vi "POST Measurement Details.vi"(0 "GTron in":path, 3 "error in":errorcluster) -> (6 "IsEmpty":bool, 9 "error out":errorcluster)   [LabVIEW 2019, in "DataLogger.lvclass"]
doc: "POST Measurement Details"
uses:
  DataLogger.lvclass
  <vilib>/drjdpowell/SQLite Library/SQL Connection/Execute SQL (Single Integer).vi
  <vilib>/httpClient/LabVIEWHTTPClient.lvlib
  <vilib>/httpClient/POSTBuffer.vi
  <vilib>/drjdpowell/SQLite Library/SQL Connection/Execute SQL (No results).vi
  <vilib>/drjdpowell/SQLite Library/SQL Statement/SQL Statement.lvclass
  <vilib>/drjdpowell/SQLite Library/SQL Connection/Open (path).vi
  <vilib>/drjdpowell/SQLite Library/SQL Connection/Connection.lvclass
panel:
  in  "Server info Cluster for Measurement in":T1={"JSON Buffer"="authtoken=47244d7c61d7e6141acdddeabbf622d1&scope=creatorapi&zc_ownername=zentron3&XMLString=", "Server information start tag"="<ZohoCreator> <applicationlist> <application name='iiot-gtron'><formlist>  <form name='SimulatedMeasurementDetails'>", "Record start/end"="add", "Key name"="field name", "Value name"="value", "Server information end tag"="\"</form></formlist></application></applicationlist></ZohoCreator>"}
  in  "Measurement Keys in":string[](array[string])=["BatchId", "PartName", "MeasurementName", "LSL", "USL", "NominalValue", "LCL", "UCL", "Mean", "StandardDeviation", "Variance", "Cp", "Cpk"]
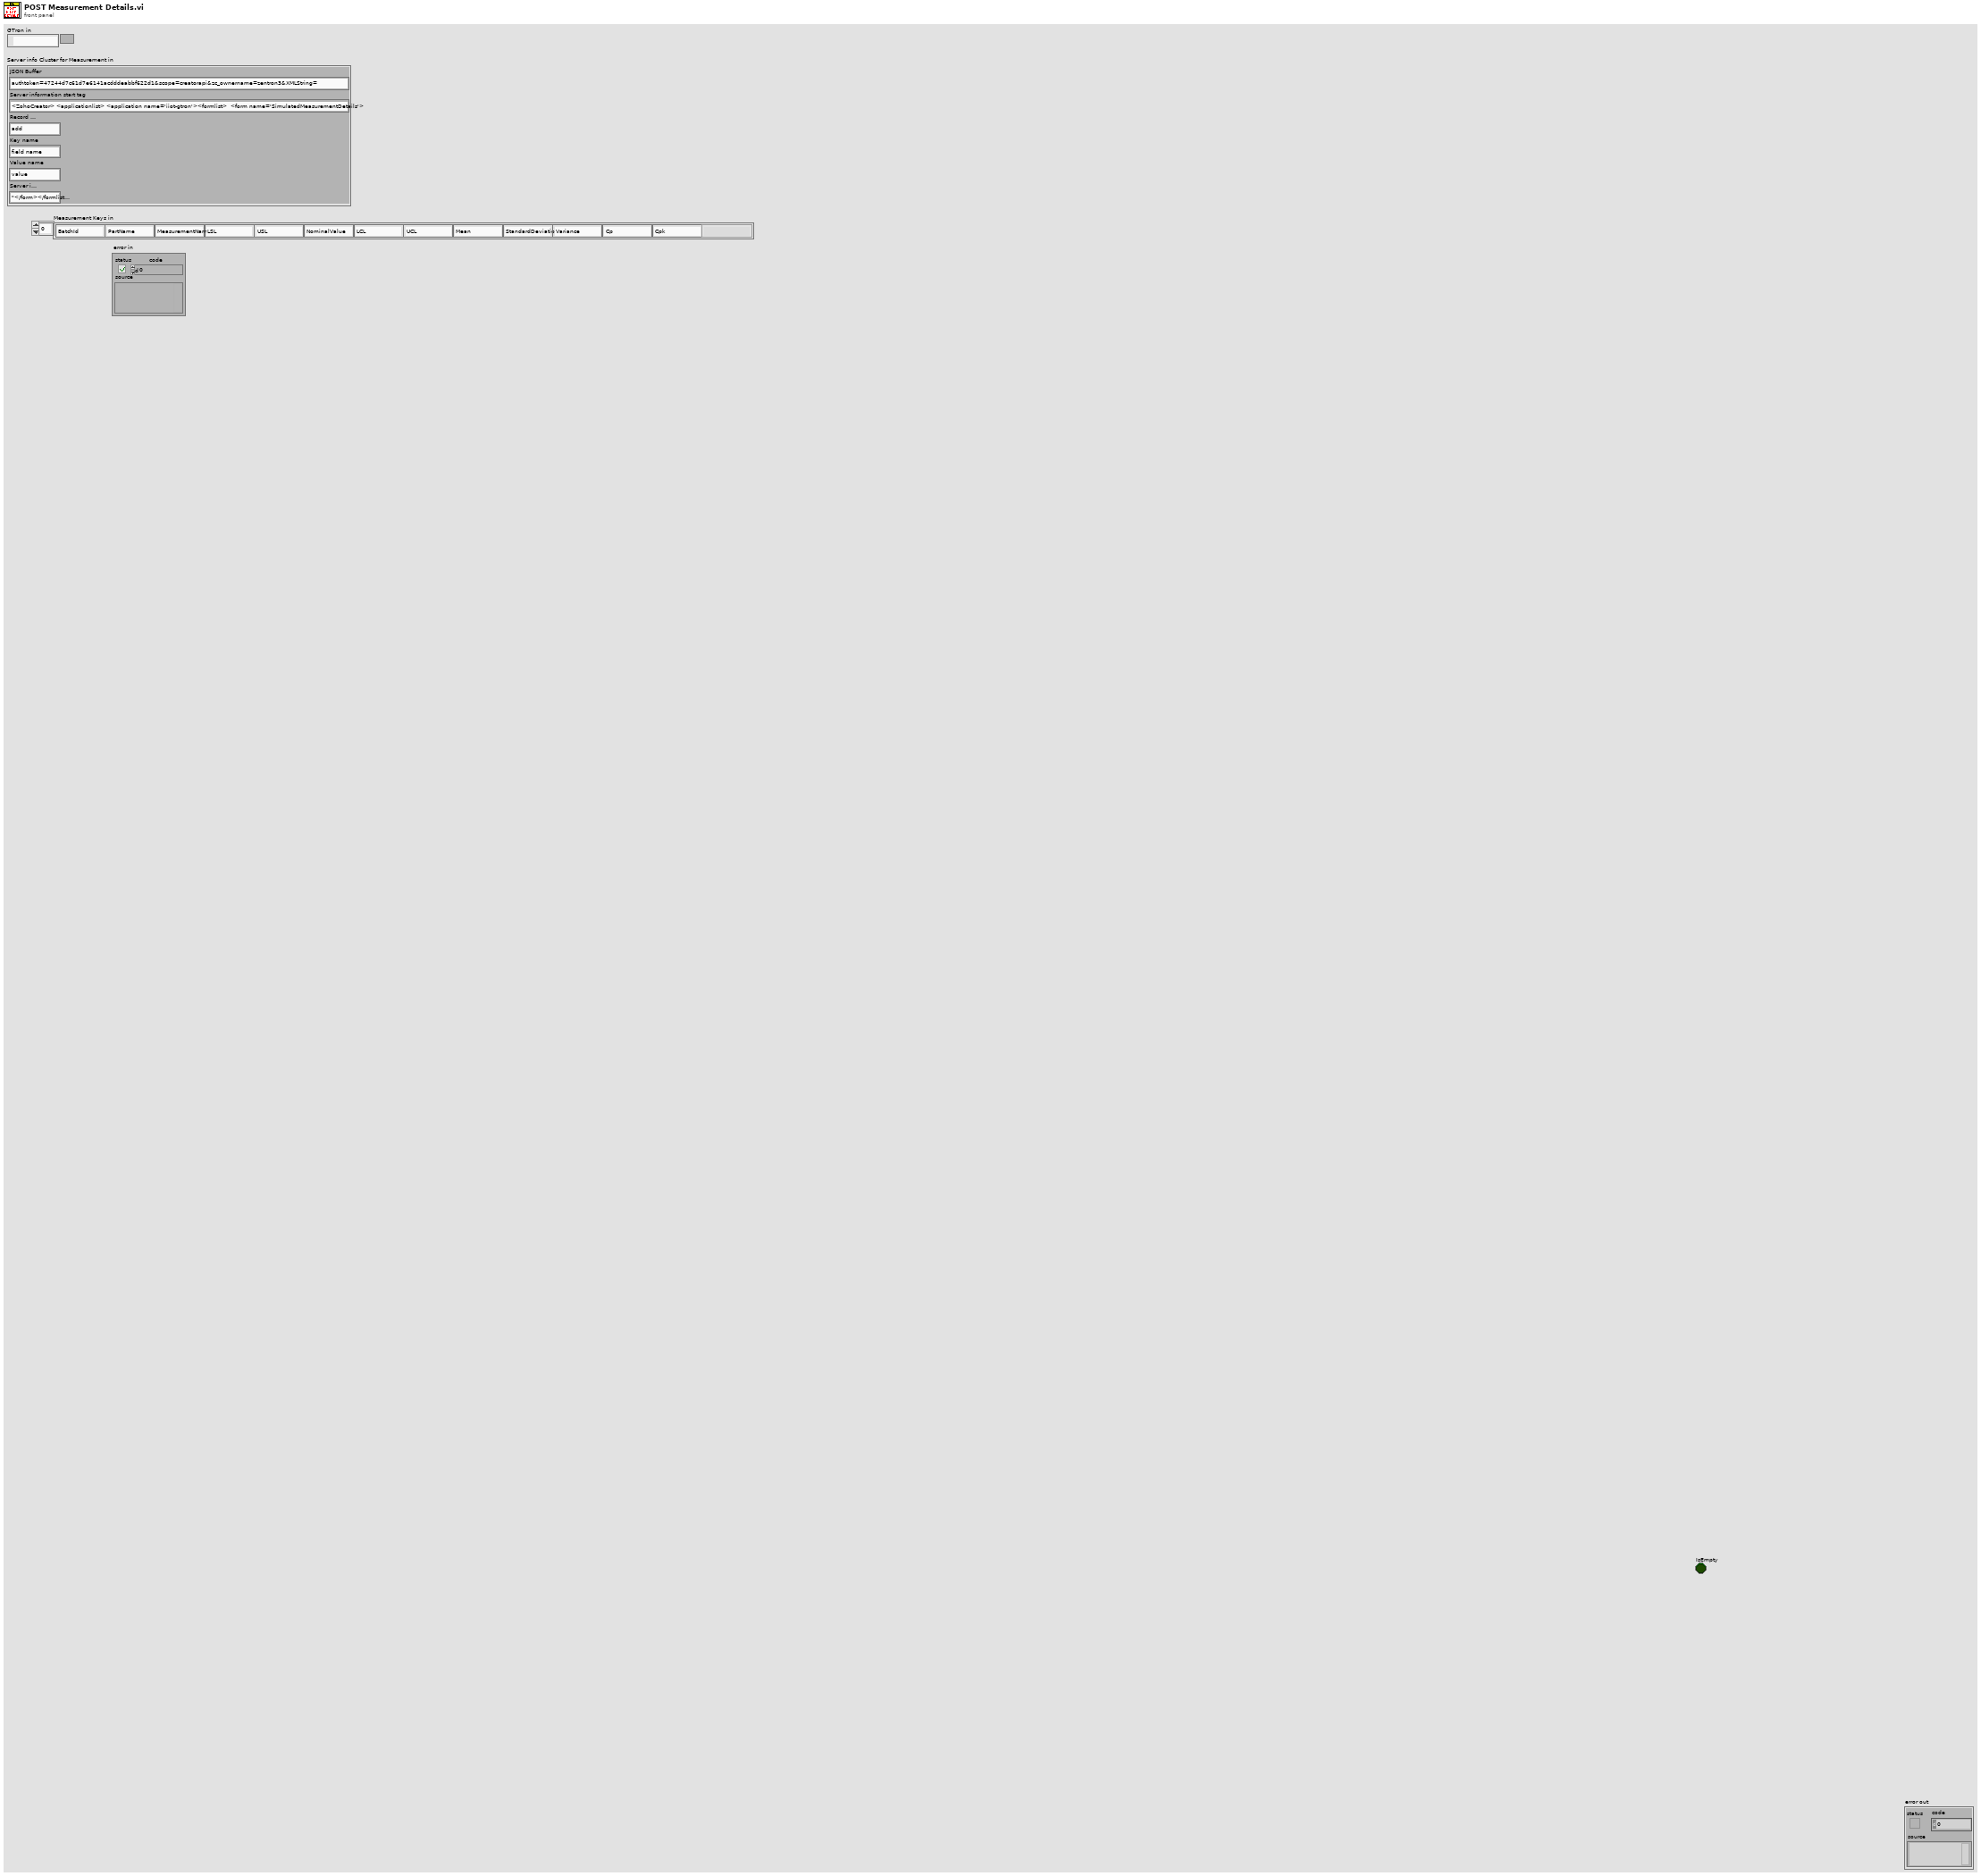
[diagram p1: front panel]
types:
  T1 = cluster{"JSON Buffer":string, "Server information start tag":string, "Record start/end":string, "Key name":string, "Value name":string, "Server information end tag":string}
  T2 = typedef "LabVIEWHTTPClient.lvlib/ClientHandle.ctl" = refnum<k1>
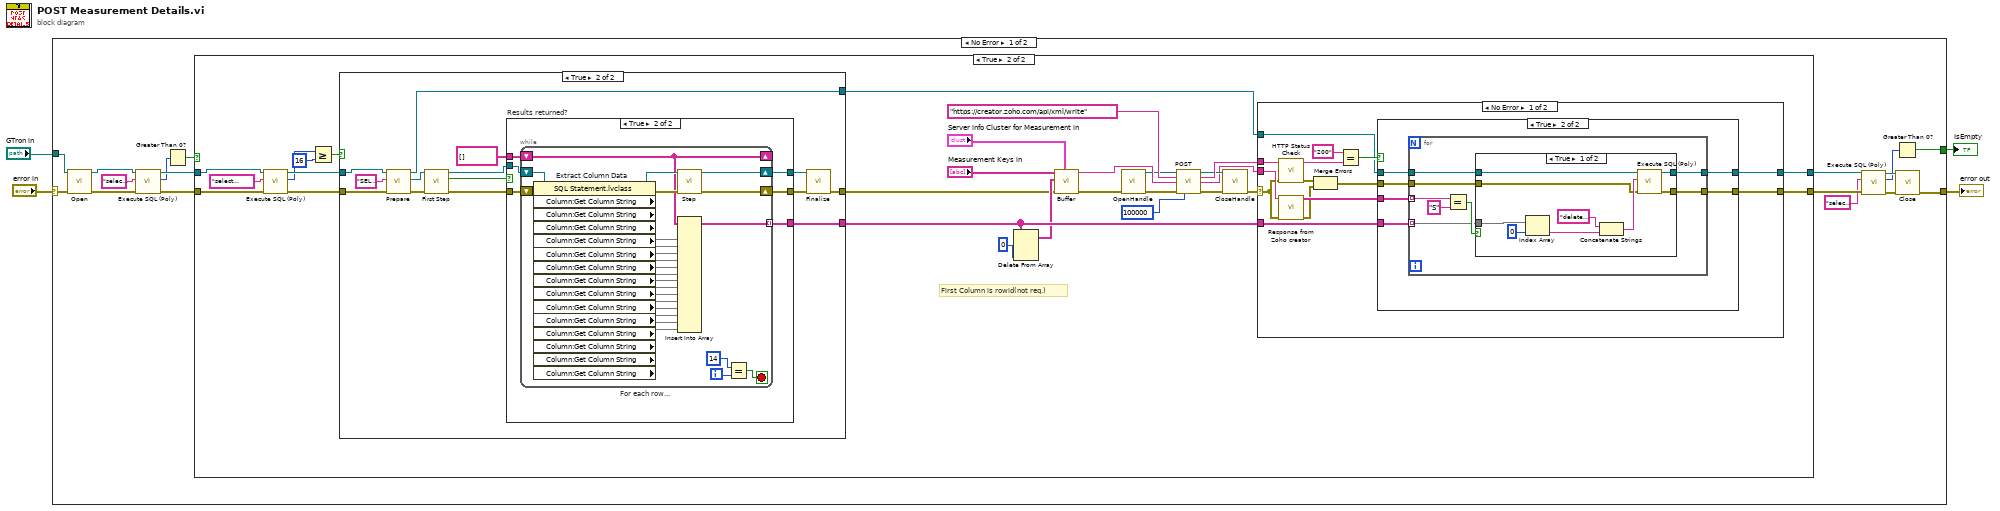
[diagram p0: block diagram]
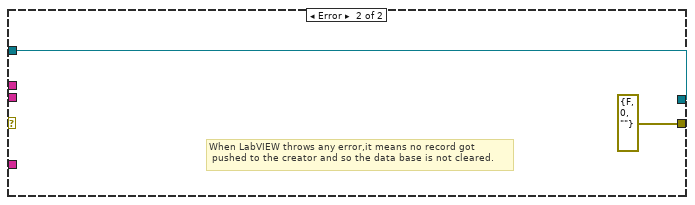
[diagram p5: hidden frame]
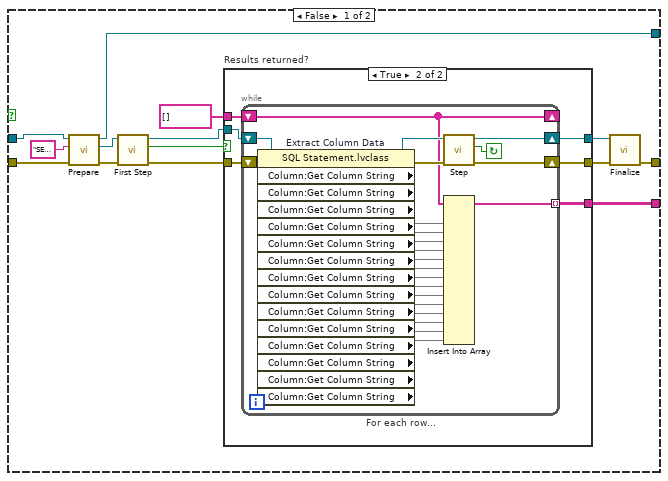
[diagram p6: hidden frame]
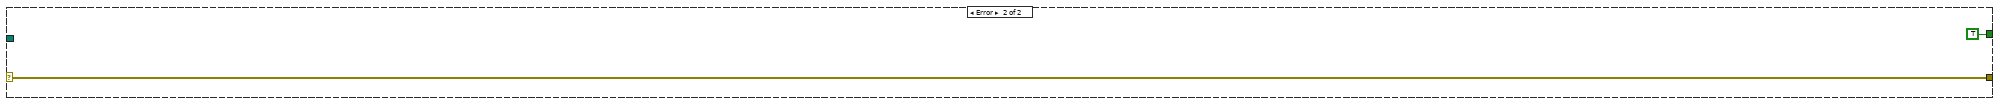
[diagram p9: hidden frame]
diagram:
  n1 = case shown="No Error" "error in" {
    selector: "error in" -> [w15 w188]
    tunnel: "GTron in" -> [w21 _]
    tunnel: [w9 w188] -> w3
    tunnel: [w6 TRUE] -> w1
    frame No Error {
      n2 = call-poly <vilib>:"Open.vi"("error in (no error)"=w15, "db file"=w21) -> ("error out"=w18:errorcluster, "SQLite Connection"=w19:refnum<class "Connection.lvclass">)  [unwired: 8 in]
      n3 = call-poly <vilib>:"Execute SQL (Poly).vi"("error in (no error)"=w18, "SQL"="select count(*) from MeasurementDetails ", "SQLite Connection in"=w19) -> ("error out"=w16:errorcluster, "Result"=w13:i64, "SQLite Connection"=w17:refnum<class "Connection.lvclass">)  [unwired: 6 in]
      n4 = Greater Than 0?(x=w13) -> (x > 0?=w14:bool)
      n5 = case shown="True" w14 {
        tunnel: w17 -> [w23 w27]
        tunnel: w16 -> [w22 w26]
        tunnel: [w23 w25] -> w7
        tunnel: [w22 w24] -> w8
        frame False {
        }
        frame True {
          # "First Column is rowid(not req.)"
          n6 = call-poly <vilib>:"Execute SQL (Poly).vi"("error in (no error)"=w26, "SQL"="select count(*) from MeasurementDetails ", "SQLite Connection in"=w27) -> ("error out"=w31:errorcluster, "Result"=w33:i64, "SQLite Connection"=w49:refnum<class "Connection.lvclass">)  [unwired: 6 in]
          n7 = Greater Or Equal?(x=w33, y=i64 16) -> (x >= y?=w35:bool)
          n8 = case shown="True" w35 {
            tunnel: [w100 w145] -> w51
            tunnel: w49 -> [w99 w144]
            tunnel: [w98 w143] -> w50
            tunnel: w31 -> [w96 w141]
            tunnel: [w95 w140] -> w30
            frame False {
              n9 = call <vilib>:"Prepare.vi"("error in (no error)"=w96, "SQL"="SELECT rowid,BatchId,PartName,MeasurementName,LSL,USL,NominalValue,LCL,UCL,Mean,StandardDeviation,Variance,Cp,Cpk FROM MeasurementDetails" ("SELECT  statement"), "SQLite Connection in"=w99) -> ("error out"=w107:errorcluster, "SQL Statement"=w103:refnum<class "SQL Statement.lvclass">, "SQLite Connection"=w98:refnum<class "Connection.lvclass">)  [unwired: 4 in, 2 out]
              n10 = call <vilib>:"First Step.vi"("error in (no error)"=w107, "SQL Statement in"=w103) -> ("error out"=w105:errorcluster, "Row returned"=w106:bool, "SQL Statement"=w104:refnum<class "SQL Statement.lvclass">)  [unwired: 7 in]
              n11 = case "Results returned?" shown="True" w106 {
                tunnel: [w110 w116] -> w102
                tunnel: [w109 w115] -> w101
                tunnel: w104 -> [w110 w114]
                tunnel: w105 -> [w109 w113]
                tunnel: string[] [] -> [_ w112]
                tunnel: [_ w111] -> w100
                frame False {
                }
                frame True {
                  n12 = while "For each row..." {
                    shift-right: [w138] -> w116
                    shift-left: w114 -> [w135]
                    shift-right: [w136] -> w115
                    shift-left: w113 -> [w134]
                    shift-right: [w133] -> _
                    shift-left: w112 -> [w133]
                    tunnel: [w125] -> w111 mode=indexing
                    stop <- w123 continue-if-true
                    n13 = property on="Extract Column Data" class="SQL Statement.lvclass"(reference=w135, error in=w134) -> (reference out=w139:refnum<class "SQL Statement.lvclass">, error out=w137:errorcluster, "Column:Get Column String"=w124, "Column:Get Column String"=w132, "Column:Get Column String"=w131, "Column:Get Column String"=w130, "Column:Get Column String"=w129, "Column:Get Column String"=w128, "Column:Get Column String"=w127, "Column:Get Column String"=w126, "Column:Get Column String"=w122, "Column:Get Column String"=w121, "Column:Get Column String"=w120, "Column:Get Column String"=w119, "Column:Get Column String"=w118, "Column:Get Column String"=w117)
                    n14 = call <vilib>:"Step.vi"("error in (no error)"=w137, "SQL Statement in"=w139) -> ("error out"=w136:errorcluster, "Row returned"=w123:bool, "SQL Statement"=w138:refnum<class "SQL Statement.lvclass">)  [unwired: 7 in]
                    n15 = Insert Into Array(array=w133, new element #1=w124, new element #2=w132, new element #3=w131, new element #4=w130, new element #5=w129, new element #6=w128, new element #7=w127, new element #8=w126, new element #9=w122, new element #10=w121, new element #11=w120, new element #12=w119, new element #13=w118, new element #14=w117) -> (w125:string[])  [unwired: 1 in]
                  }
                }
              }
              n16 = call <vilib>:"Finalize.vi"("error in (no error)"=w101, "SQL Statement in"=w102) -> ("error out"=w95:errorcluster)  [unwired: 9 in]
            }
            frame True {
              n17 = call <vilib>:"Prepare.vi"("error in (no error)"=w141, "SQL"="SELECT rowid,BatchId,PartName,MeasurementName,LSL,USL,NominalValue,LCL,UCL,Mean,StandardDeviation,Variance,Cp,Cpk FROM MeasurementDetails" ("SELECT  statement"), "SQLite Connection in"=w144) -> ("error out"=w152:errorcluster, "SQL Statement"=w148:refnum<class "SQL Statement.lvclass">, "SQLite Connection"=w143:refnum<class "Connection.lvclass">)  [unwired: 4 in, 2 out]
              n18 = call <vilib>:"First Step.vi"("error in (no error)"=w152, "SQL Statement in"=w148) -> ("error out"=w150:errorcluster, "Row returned"=w151:bool, "SQL Statement"=w149:refnum<class "SQL Statement.lvclass">)  [unwired: 7 in]
              n19 = case "Results returned?" shown="True" w151 {
                tunnel: [w155 w161] -> w147
                tunnel: [w154 w160] -> w146
                tunnel: w149 -> [w155 w159]
                tunnel: w150 -> [w154 w158]
                tunnel: string[] [] -> [_ w157]
                tunnel: [_ w156] -> w145
                frame False {
                }
                frame True {
                  n20 = while "For each row..." {
                    shift-right: [w185] -> w161
                    shift-left: w159 -> [w182]
                    shift-right: [w183] -> w160
                    shift-left: w158 -> [w181]
                    shift-right: [w180] -> _
                    shift-left: w157 -> [w180]
                    tunnel: [w172] -> w156 mode=indexing
                    i -> [w171]
                    stop <- w169 stop-if-true
                    n21 = property on="Extract Column Data" class="SQL Statement.lvclass"(reference=w182, error in=w181) -> (reference out=w186:refnum<class "SQL Statement.lvclass">, error out=w184:errorcluster, "Column:Get Column String"=w168, "Column:Get Column String"=w179, "Column:Get Column String"=w178, "Column:Get Column String"=w177, "Column:Get Column String"=w176, "Column:Get Column String"=w175, "Column:Get Column String"=w174, "Column:Get Column String"=w173, "Column:Get Column String"=w167, "Column:Get Column String"=w166, "Column:Get Column String"=w165, "Column:Get Column String"=w164, "Column:Get Column String"=w163, "Column:Get Column String"=w162)
                    n22 = call <vilib>:"Step.vi"("error in (no error)"=w184, "SQL Statement in"=w186) -> ("error out"=w183:errorcluster, "SQL Statement"=w185:refnum<class "SQL Statement.lvclass">)  [unwired: 7 in, 1 out]
                    n23 = Insert Into Array(array=w180, new element #1=w168, new element #2=w179, new element #3=w178, new element #4=w177, new element #5=w176, new element #6=w175, new element #7=w174, new element #8=w173, new element #9=w167, new element #10=w166, new element #11=w165, new element #12=w164, new element #13=w163, new element #14=w162) -> (w172:string[])  [unwired: 1 in]
                    n24 = Equal?(x=14, y=w171) -> (x = y?=w169:bool)
                  }
                }
              }
              n25 = call <vilib>:"Finalize.vi"("error in (no error)"=w146, "SQL Statement in"=w147) -> ("error out"=w140:errorcluster)  [unwired: 9 in]
            }
          }
          n26 = Delete From Array(array=w51, index (col)=0 ("disabled index (col)")) -> (array with subset deleted=w37:string[][])  [unwired: 2 in, 1 out]
          n27 = call "Buffer.vi"("Cluster"="Server info Cluster for Measurement in", "error in"=w30, "Values"=w37, "Keys"="Measurement Keys in") -> ("Error out"=w29:errorcluster, "Buffer"=w42:string)  [unwired: 6 in]
          n28 = call <vilib>:"OpenHandle.vi"("error in (no error)"=w29) -> ("client handle out"=w40:T2, "error out"=w45:errorcluster)  [unwired: 13 in]
          n29 = call-poly <vilib>:"POST.vi"("client handle"=w40, "url"="https://creator.zoho.com/api/xml/write", "buffer"=w42, "error in (no error)"=w45, "timeout (10000)"=100000) -> ("client handle out"=w41:T2, "headers"=w48:string, "body"=w28:string, "error out"=w46:errorcluster)  [unwired: 7 in]
          n30 = call <vilib>:"CloseHandle.vi"("client handle"=w41, "error in (no error)"=w46) -> ("error out"=w47:errorcluster)  [unwired: 13 in]
          n31 = case shown="No Error" w47 {
            selector: w47 -> [w56 _]
            tunnel: w48 -> [w65 _]
            tunnel: w28 -> [w58 _]
            tunnel: w50 -> [w61 w94]
            tunnel: w51 -> [w60 _]
            tunnel: [w59 w94] -> w25
            tunnel: [w52 errorcluster {"status"=FALSE, "code"=0, "source"=""} ("error out")] -> w24
            frame No Error {
              n32 = call "HTTP Status Check.vi"("error in (no error)"=w56, "String"=w65) -> ("error out"=w55:errorcluster, "HTTP Status Code"=w64:string)  [unwired: 7 in]
              n33 = call "Response from Zoho creator.vi"("error in"=w56, "body"=w58) -> ("error out"=w54:errorcluster, "decimated array"=w57:string[])  [unwired: 8 in]
              n34 = Merge Errors(w55, w54) -> (w53:errorcluster)
              n35 = Equal?(x="200" ("y"), y=w64) -> (x = y?=w62:bool)
              n36 = case shown="True" w62 {
                tunnel: w57 -> [_ w72]
                tunnel: w61 -> [w67 w73]
                tunnel: w60 -> [_ w71]
                tunnel: [w67 w70] -> w59
                tunnel: w53 -> [w66 w69]
                tunnel: [w66 w68] -> w52
                frame False {
                  # "When HTTP Status is anything except 200,it means no record\ngot pushed to the creator and so the database is not cleared"
                }
                frame True {
                  n37 = for {
                    tunnel: w73 -> [w81]
                    tunnel: w71 -> [w77] mode=indexing
                    tunnel: w72 -> [w80] mode=indexing
                    tunnel: [w76] -> w70
                    tunnel: w69 -> [w75]
                    tunnel: [w74] -> w68
                    n38 = Equal?(x=w80, y="S") -> (x = y?=w78:bool)
                    n39 = case shown="True" w78 {
                      tunnel: w81 -> [w90 w92]
                      tunnel: w77 -> [w89 _]
                      tunnel: [w84 w92] -> w76
                      tunnel: w75 -> [w83 w91]
                      tunnel: [w82 w91] -> w74
                      frame True {
                        n40 = Index Array(array=w89, index=0) -> (element=w87:string)
                        n41 = Concatenate Strings("delete from MeasurementDetails where rowid = " ("SQL"), w87) -> (w85:string)
                        n42 = call-poly <vilib>:"Execute SQL (Poly).vi"("error in (no error)"=w83, "SQL"=w85, "SQLite Connection in"=w90) -> ("error out"=w82:errorcluster, "SQLite Connection"=w84:refnum<class "Connection.lvclass">)  [unwired: 7 in]
                      }
                      frame False {
                      }
                    }
                  }
                }
              }
            }
            frame Error {
              # "When LabVIEW throws any error,it means no record got\n pushed to the creator and so the data base is not cleared."
            }
          }
        }
      }
      n43 = call-poly <vilib>:"Execute SQL (Poly).vi"("error in (no error)"=w8, "SQL"="select count(*) from MeasurementDetails ", "SQLite Connection in"=w7) -> ("error out"=w12:errorcluster, "Result"=w10:i64, "SQLite Connection"=w11:refnum<class "Connection.lvclass">)  [unwired: 6 in]
      n44 = Greater Than 0?(x=w10) -> (x > 0?=w6:bool)
      n45 = call-dynamic "Close.vi"("error in (no error)"=w12, "SQLite Connection in"=w11) -> ("error out"=w9:errorcluster)  [unwired: 9 in]
    }
    frame Error {
    }
  }
  "error out" <- w3
  "IsEmpty" <- w1
